vi "getSpectrumFromFile.vi"(11 "File Path Control":path) -> (2 "array":dbl[][](array[numeric]))   [LabVIEW 2022 SP3]
panel:
  out "error out":errorcluster
  out "The Data":string
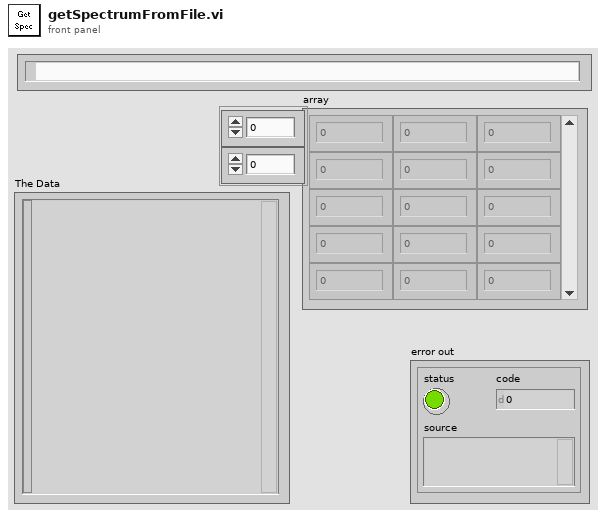
[diagram p1: front panel]
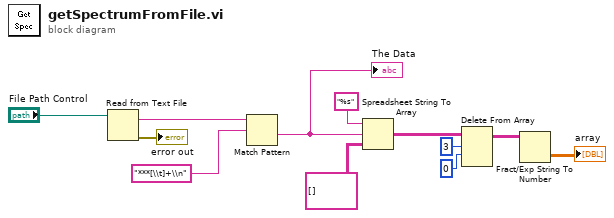
[diagram p0: block diagram]
diagram:
  n1 = Read from Text File(file (use dialog)="File Path Control") -> (text=w7:string, error out=→"error out":errorcluster)  [unwired: 3 in, 2 out]
  n2 = Match Pattern(string=w7, regular expression="***[\\t]+\\n" ("end of header")) -> (after substring=w8:string)  [unwired: 1 in, 3 out]
  "The Data" <- w8
  n3 = Spreadsheet String To Array(format string="%s", spreadsheet string=w8, array type (2D Dbl)=string[][] []) -> (array=w5:string[][])  [unwired: 1 in]
  n4 = Delete From Array(array=w5, length=3, index (row)=0) -> (array with subset deleted=w2:string[][])  [unwired: 1 in, 1 out]
  n5 = Fract/Exp String To Number(string=w2) -> (number=→"array":dbl[][])  [unwired: 3 in, 1 out]
